vi "ClusterwitharrayCEXT.vi"(1 "Cluster In":cluster{"Array In":cxt[], "Numeric Input":cxt} {"Numeric Input" format="%.2f"; "Array In" format="%.2f"}, 2 "Base":cxt format="%.2f") -> (0 "Cluster Out":cluster{"Array Out":cxt[], "Numeric Output":cxt} {"Numeric Output" format="%.2f"; "Array Out" format="%.2f"})   [LabVIEW 2010]
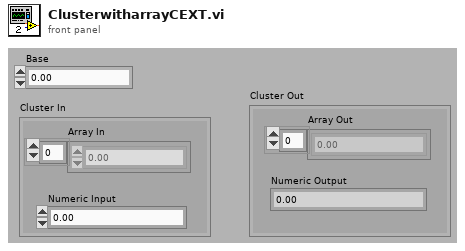
[diagram p1: front panel]
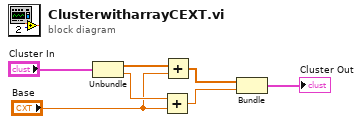
[diagram p0: block diagram]
diagram:
  n1 = Unbundle("Cluster In") -> ("Array In"=w7:cxt[], "Numeric Input"=w6:cxt)
  n2 = Add(x=w6, y="Base") -> (x+y=w4:cxt)
  n3 = Add(x=w7, y="Base") -> (x+y=w5:cxt[])
  n4 = Bundle(w5, w4) -> (→"Cluster Out":cluster{cxt[], cxt})  [unwired: 1 out]
